vi "clearpath_message_parser.vi"(1 "Input Array":u8[](array[numeric]) format="%x") -> (2 "Payload":u8[](array[numeric]) format="%x", 3 "Timestamp":u32 format="%x", 4 "Message Length":u16, 5 "Message Type":u16 format="%x", 6 "Checksum Valid":bool)   [LabVIEW 2012, in "clearpath_interface.lvlib"]
doc: "Provides access to the properties of a CCP message"
uses:
  clearpath_interface.lvlib
  cwrap_crio.dll
panel:
  out "Calculated Checksum":u16 format="%x"
  out "Message Checksum":u16 format="%x"
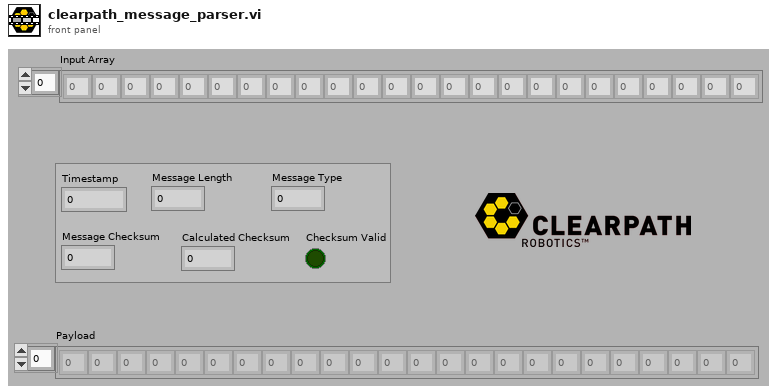
[diagram p1: front panel]
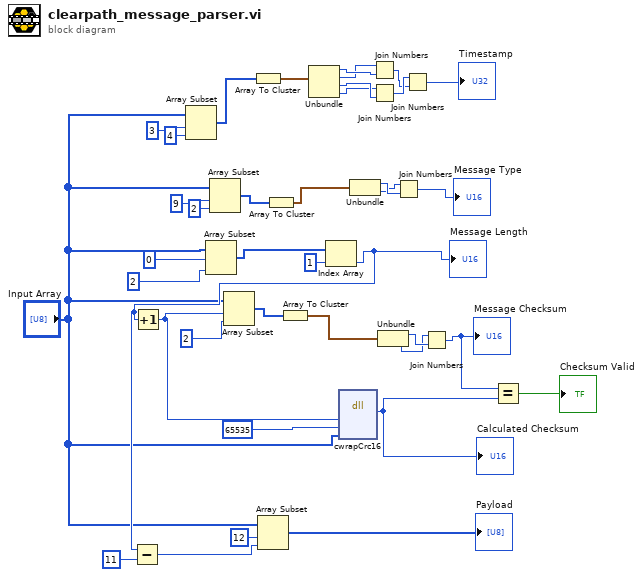
[diagram p0: block diagram]
diagram:
  n1 = Array Subset(array="Input Array", index=3, length=4) -> (w36:u8[])
  n2 = Array Subset(array="Input Array", index=0, length=2) -> (w23:u8[])
  n3 = Array Subset(array="Input Array", index=9, length=2) -> (w31:u8[])
  n4 = Array To Cluster(array=w36) -> (cluster=w35:cluster{"[0]":u8, "[1]":u8, "[2]":u8, "[3]":u8})
  n5 = Array To Cluster(array=w31) -> (cluster=w30:cluster{"[0]":u8, "[1]":u8})
  n6 = Unbundle(w35) -> ("[0]"=w10:u8, "[1]"=w9:u8, "[2]"=w8:u8, "[3]"=w7:u8)
  n7 = Index Array(array=w23, index=1) -> (element=w15:u8)
  "Message Length" <- w15
  n8 = Subtract(x=w15, y=u8 11) -> (x-y=w14:u8)
  n9 = Increment(x=w15) -> (x+1=w6:u8)
  n10 = Array Subset(array="Input Array", index=w6, length=2) -> (w27:u8[])
  n11 = Array Subset(array="Input Array", index=12, length=w14) -> (→"Payload":u8[])
  n12 = Array To Cluster(array=w27) -> (cluster=w26:cluster{"[0]":u8, "[1]":u8})
  n13 = dll-call lib="C:/Users/tebbeam/Documents/GitHub/IGVC-2013/Code/Project 1.0/Motors/Husky/cwrap_cRIO.*" fn="cwrapCrc16"("size"=w6, "init_val"=65535, "data"="Input Array") -> ("return type"=w1:u16)  [unwired: 6 in, 2 out]
  "Calculated Checksum" <- w1
  n14 = Unbundle(w30) -> ("[0]"=w21:u8, "[1]"=w20:u8)
  n15 = Join Numbers(hi=w9, lo=w10) -> ((hi.lo)=w11:u16)
  n16 = Join Numbers(hi=w7, lo=w8) -> ((hi.lo)=w12:u16)
  n17 = Unbundle(w26) -> ("[0]"=w19:u8, "[1]"=w18:u8)
  n18 = Join Numbers(hi=w20, lo=w21) -> ((hi.lo)=→"Message Type":u16)
  n19 = Join Numbers(hi=w12, lo=w11) -> ((hi.lo)=→"Timestamp":u32)
  n20 = Join Numbers(hi=w18, lo=w19) -> ((hi.lo)=w2:u16)
  "Message Checksum" <- w2
  n21 = Equal?(x=w2, y=w1) -> (x = y?=→"Checksum Valid":bool)
